vi "AMX-CCD2 自动处理图像.vi"(0 "Image In":T1(plugin-control), 5 "名称或相对路径":string="Template Program", 11 "error in (no error)":errorcluster caption="错误输入（无错误）") -> (4 "Image Out":T1(plugin-control), 6 "NO LINES":bool, 8 "CCD2-L":bool, 10 "CCD2-R":bool, 15 "error out":errorcluster caption="错误输出")   [LabVIEW 2017]
uses:
  Global System.vi
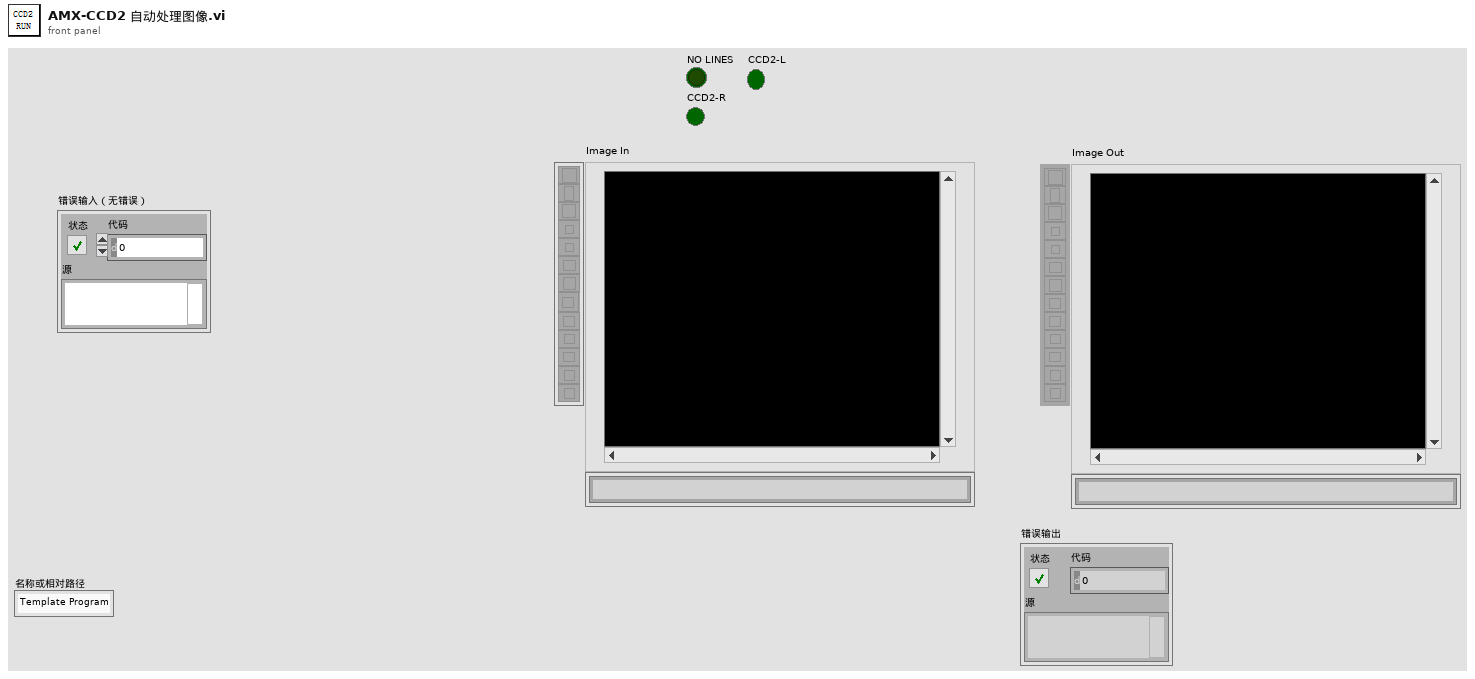
[diagram p1: front panel]
types:
  T1 = typedef "IMAQ Image.ctl" = refnum<image>
  T2 = typedef "IMAQ Rectangle" = cluster{"Left":i32, "Top":i32, "Right":i32, "Bottom":i32, "Rotation":dbl}
  T3 = typedef "IMAQ Curve Parameters.ctl" = cluster{"Extraction Mode":u32, "Edge Threshold":i32, "Edge Filter Size":u32, "Min Length":i32, "Row Search Step Size":i32, "Col Search Step Size":i32, "Max Endpoint Gap":i32, "Closed":bool, "Subpixel":bool}
  T4 = cluster{"Rectangle":T2, "Angle (degrees) ":sgl, "long":sgl, "abgek":dbl, "Color":u32, "left threshold":dbl, "Rectangle right":T2, "long right":sgl, "abgek right":dbl, "Color 2":u32, "right threshold":dbl, "left":dbl, "right":dbl, "Settings (Big)":T3, "Clamp Settings (Big)":cluster{"Angle ":dbl, "Edge Polarity":cluster{"Start":u32, "End":u32}}, " Settings top":T3, "Clamp Settings top ":cluster{"Angle ":dbl, "Edge Polarity":cluster{"Start":u32, "End":u32}}, "Sub-Pixel Accuracy ":bool, "Threshold Parameters":cluster{"Level Type":enum32{"Absolute Value", "Relative value"}, "Threshold Level":i32, "Hysteresis":i32}, "Process ":enum16{"Get First Edge", "Get First + Last Edge", "Get All Edges"}, "Threshold Parameters 2":cluster{"Level Type":enum32{"Absolute Value", "Relative value"}, "Threshold Level":i32, "Hysteresis":i32}}
  T5 = typedef "IMAQ Line" = cluster{"Start X":i32, "Start Y":i32, "End X":i32, "End Y":i32}
  T6 = cluster{"Rectangle big CCD1":T2, "Rectangle top CCD1 ":T2, "Line":T5, "left line ":dbl, "right line":dbl}
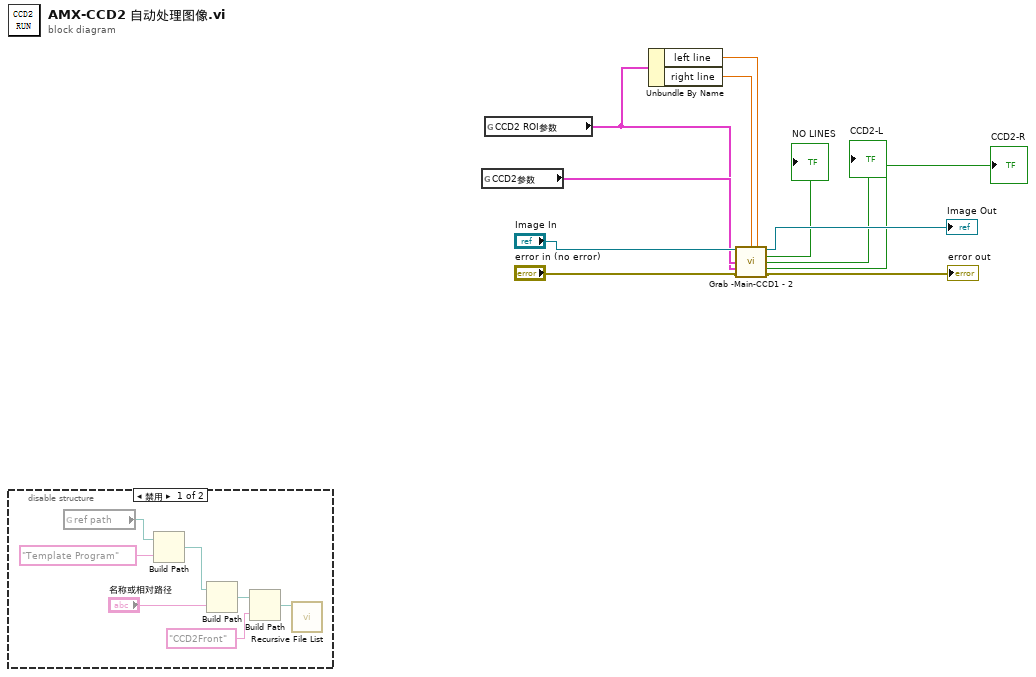
[diagram p0: block diagram]
diagram:
  n1 = disable-structure shown="禁用" {
    frame Disabled {
      n2 = global read "Global System.vi" "ref path"() -> (w17:path)
      n3 = Build Path(base path=w17, name or relative path="Template Program" ("名称或相对路径")) -> (appended path=w15:path)
      n4 = Build Path(base path=w15, name or relative path="名称或相对路径") -> (appended path=w12:path)
      n5 = Build Path(base path=w12, name or relative path="CCD2Front" ("名称或相对路径")) -> (appended path=w13:path)
      n6 = call <vilib>:"Recursive File List.vi"("Folder Path"=w13) -> ()  [unwired: 6 in, 5 out]
    }
    frame Enabled {
    }
  }
  n7 = global read "Global System.vi" "CCD2参数"() -> (w4:T4)
  n8 = global read "Global System.vi" "CCD2 ROI参数"() -> (w3:T6)
  n9 = Unbundle By Name(w3) -> ("left line"=w2:dbl, "right line"=w1:dbl)
  n10 = call "Grab -Main-CCD1 - 2.vi"("Image in"="Image In", "right"=w1, "left"=w2, "CCD2参数"=w4, "ROI参数"=w3, "error in (no error)"="error in (no error)") -> ("Image out"=→"Image Out":T1, "NO LINES"=→"NO LINES":bool, "CCD2-L"=→"CCD2-L":bool, "CCD2-R"=→"CCD2-R":bool, "error out"=→"error out":errorcluster)  [unwired: 5 in]
